vi "Create Session.vi"(8 "error in (no error)":errorcluster, 11 "Session Id":u64) -> (0 "error out":errorcluster, 1 "Run Time Configuration":string, 2 "Edit Time Configuration":string, 3 "Session out":refnum<class "Plugin Session.lvclass">, 4 "Panel Size":T1)   [LabVIEW 2020, in "InstrumentStudio Plugin SDK.lvlib" / "Plugin Session.lvclass"]
doc: "Call this VI with the Session Id as the first SDK call at the beginning of your plugin VI. This VI sets up the events and other data needed for the plugin panel and framework to communicate. If you need to know the panel size for your plugin panel to adjust its front panel, this VI will return the size. Some plugin panels support both large and small panel sizes and need to adjust the visuals on their front panel to better fit into that panel size. LabVIEW plugin panels are uniquely identified by the Plugin Session which is set by the framework when the plugin is run. Plugins must have a control named 'Session Id' which is a U64 numeric control on their plugin VI front panel so the framework can correctly set it. This 'Session Id' is then passed to Create Session.vi to begin the plugin session. This control can be placed on the user's VI by right-clicking on the input of the Create Session.vi and choosing 'Create Control'.\nThe Plugin Session returned is then used to call other SDK VIs during execution of the plugin VI to get or set properties of the plugin panel or to notify the framework of various events."
uses:
  Plugin Session.lvclass
  Panel Size.ctl
  Plugin Events.ctl
  Event Registration Refnum.ctl
  Plugin Session.lvclass/Plugin Session.ctl
  Read Edit Time Configuration.vi
  Read Run Time Configuration.vi
  InstrumentStudio Plugin SDK.lvlib
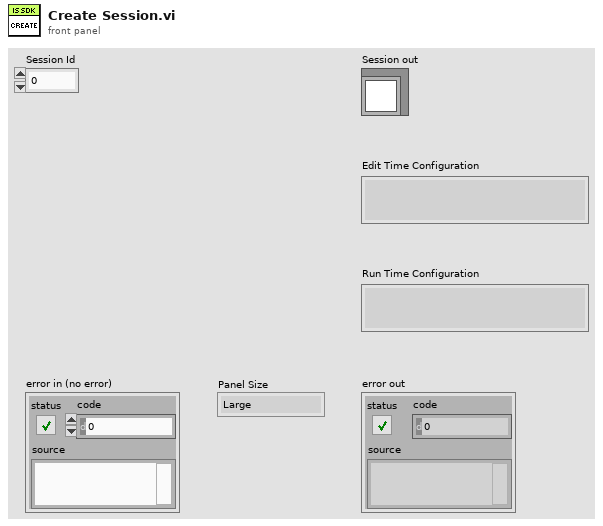
[diagram p1: front panel]
types:
  T1 = typedef "InstrumentStudio Plugin SDK.lvlib/Panel Size.ctl" = enum32{"Large", "Small"}
  T2 = typedef "InstrumentStudio Plugin SDK.lvlib/Plugin Events.ctl" = cluster{"Shutdown":refnum<user-event>, "Project Saved":refnum<user-event>, "Stop All Outputs":refnum<user-event>, "Generic Message":refnum<user-event>, "Active Pin Map Changed":refnum<user-event>, "Selected Sites Changed":refnum<user-event>}
  T3 = typedef "InstrumentStudio Plugin SDK.lvlib/Event Registration Refnum.ctl" = refnum<event-registration>
  T4 = cluster{"Session Id":u64, "Plugin Events":T2, "Event Refnum":T3}
  T5 = cluster{"Active Pin Map Path":path, "Completion Id":i64}
  T6 = cluster{"Name":string, "Data":string, "Completion Id":i64}
  T7 = cluster{"Project Path":path, "Completion Id":i64}
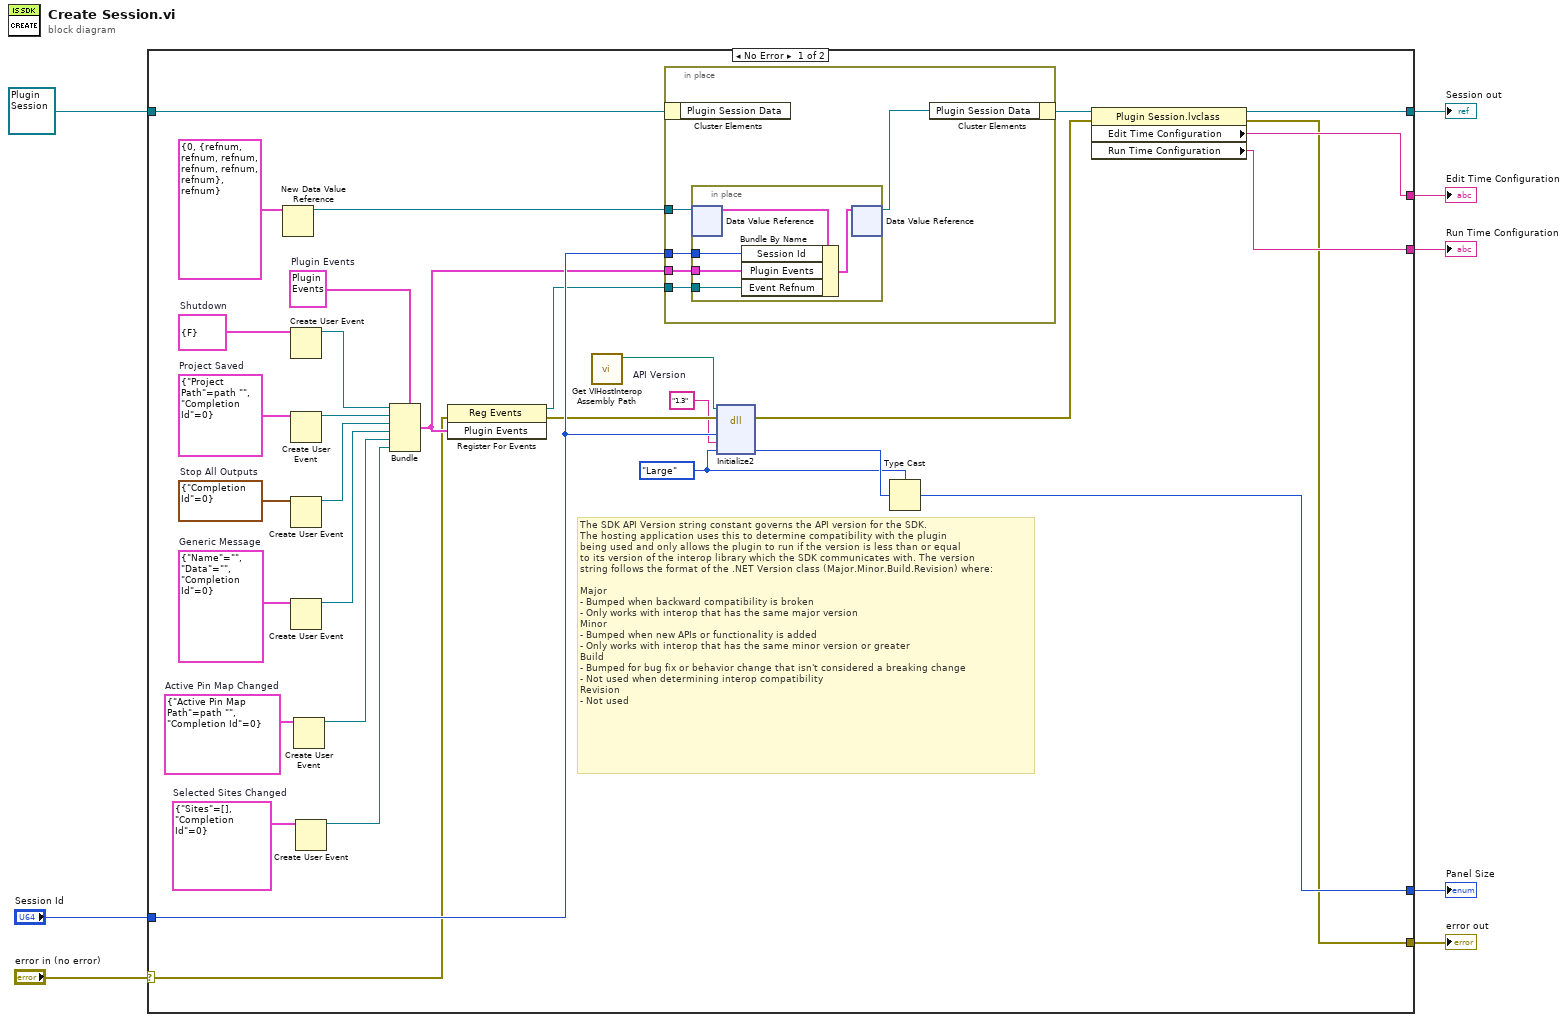
[diagram p0: block diagram]
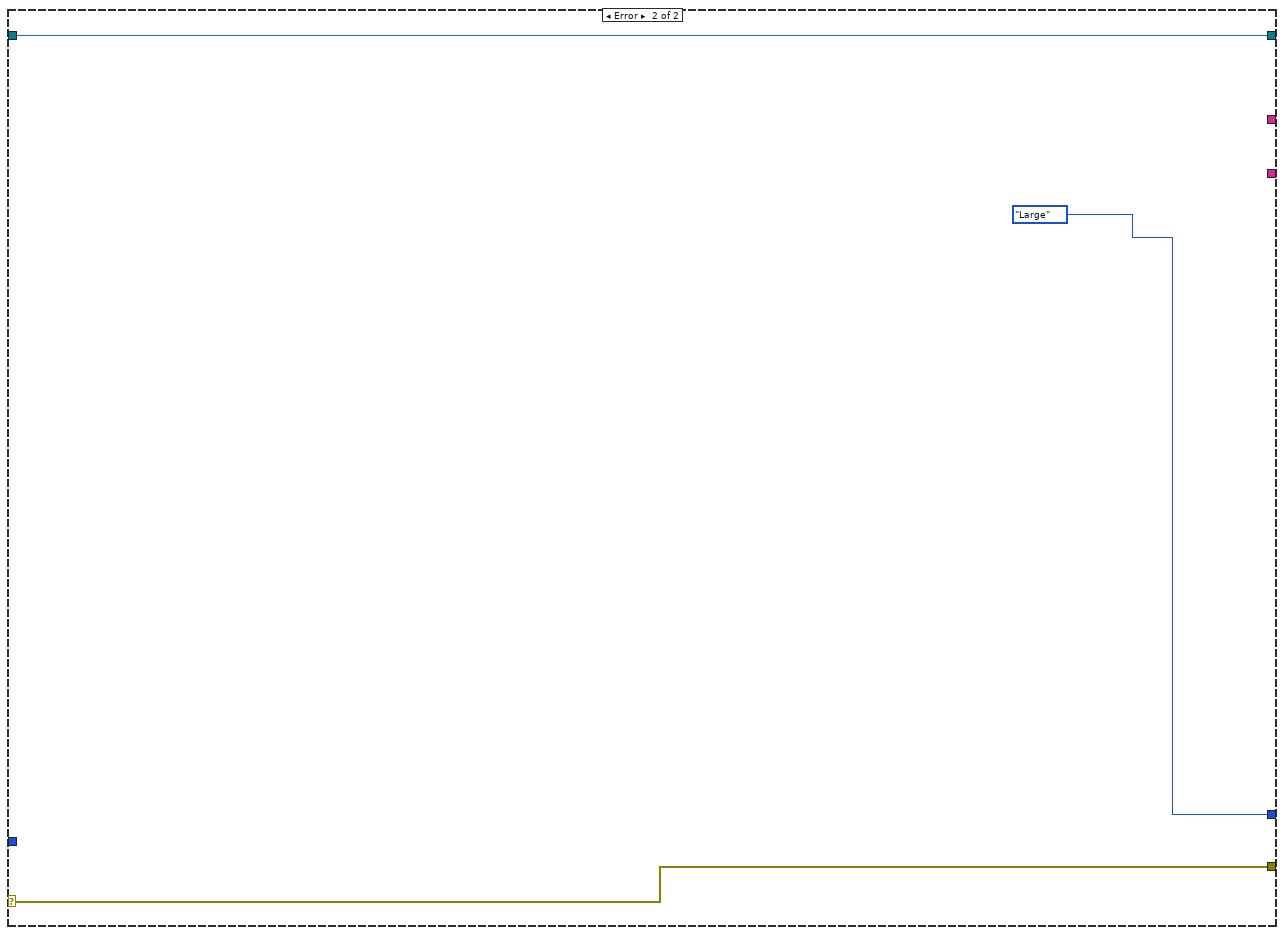
[diagram p2: hidden frame]
diagram:
  n1 = case shown="No Error" "error in (no error)" {
    selector: "error in (no error)" -> [w29 w52]
    tunnel: [w23 w52] -> w8
    tunnel: [w38 Panel_Size."Large" ("Panel Size")] -> w7
    tunnel: "Session Id" -> [w34 _]
    tunnel: refnum<class "Plugin Session.lvclass"> refnum ("PluginSDK:PluginSession.lvclass") -> [w31 w51]
    tunnel: [w24 w51] -> w3
    tunnel: [w27 _] -> w2
    tunnel: [w25 _] -> w1
    frame No Error {
      w13 = cluster{"Sites":i32[], "Completion Id":i64} {"Sites"=[], "Completion Id"=0}  # Selected Sites Changed
      w14 = T5 {"Active Pin Map Path"=path "", "Completion Id"=0}  # Active Pin Map Changed
      w15 = "1.3"  # API Version
      w17 = T6 {"Name"="", "Data"="", "Completion Id"=0}  # Generic Message
      w21 = cluster{"Unused":bool} {"Unused"=FALSE}  # Shutdown
      w12 = T2 {"Shutdown"=refnum, "Project Saved"=refnum, "Stop All Outputs"=refnum, "Generic Message"=refnum, "Active Pin Map Changed"=refnum, "Selected Sites Changed"=refnum}  # Plugin Events
      w36 = T7 {"Project Path"=path "", "Completion Id"=0}  # Project Saved
      w37 = cluster{"Completion Id":i64} {"Completion Id"=0}  # Stop All Outputs
      w39 = Panel_Size."Large" ("Panel Size")
      # "The SDK API Version string constant governs the API version for the SDK.\nThe hosting application uses this to determine compatibility with the plugin\nbeing used and only allows the plugin to run if the version is less than or equal\nto its version of the interop library which the SDK communicates with. The version\nstring follows the format of the .NET Version class (Major.Minor.Build.Revision) where:\n\nMajor\n- Bumped when backward compatibility is broken\n- Only works with interop that has the same major version\nMinor\n- Bumped when new APIs or functionality is added\n- Only works with interop that has the same minor version or greater\nBuild\n- Bumped for bug fix or behavior change that isn't considered a breaking change\n- Not used when determining interop compatibility\nRevision\n- Not used"
      n2 = New Data Value Reference(data value=T4 {"Session Id"=0, "Plugin Events"={"Shutdown"=refnum, "Project Saved"=refnum, "Stop All Outputs"=refnum, "Generic Message"=refnum, "Active Pin Map Changed"=refnum, "Selected Sites Changed"=refnum}, "Event Refnum"=refnum} ("Cluster of class private data")) -> (data value reference=w35:refnum<data-value>)  [unwired: 1 in, 1 out]
      n3 = Create User Event(user event datatype=w21) -> (user event=w20:refnum<user-event>)  [unwired: 1 in, 1 out]
      n4 = Create User Event(user event datatype=w36) -> (user event=w19:refnum<user-event>)  [unwired: 1 in, 1 out]
      n5 = Create User Event(user event datatype=w37) -> (user event=w18:refnum<user-event>)  [unwired: 1 in, 1 out]
      n6 = Create User Event(user event datatype=w17) -> (user event=w16:refnum<user-event>)  [unwired: 1 in, 1 out]
      n7 = Create User Event(user event datatype=w14) -> (user event=w11:refnum<user-event>)  [unwired: 1 in, 1 out]
      n8 = Create User Event(user event datatype=w13) -> (user event=w10:refnum<user-event>)  [unwired: 1 in, 1 out]
      n9 = Bundle(cluster=w12, "Shutdown"=w20, "Project Saved"=w19, "Stop All Outputs"=w18, "Generic Message"=w16, "Active Pin Map Changed"=w11, "Selected Sites Changed"=w10) -> (w33:T2)
      n10 = register-events(error in=w29, w33) -> (reference out=w32:refnum<event-registration>, error out=w30:errorcluster)  [unwired: 1 in]
      n11 = call "Get VIHostInterop Assembly Path.vi"() -> ("VIHost.Interop Assembly"=w9:path)  [unwired: 11 in]
      n12 = in-place {
        in-place-border: w35 -> [w45]
        in-place-border: w34 -> [w44]
        in-place-border: w33 -> [w43]
        in-place-border: w32 -> [w42]
        n13 = in-place-cluster #1(w31) -> ()  [unwired: 1 out]
        n14 = in-place {
          in-place-border: w44 -> [w49]
          in-place-border: w43 -> [w48]
          in-place-border: w42 -> [w47]
          n15 = in-place-dvr #2(w45) -> (w50:T4)  [unwired: 1 out]
          n16 = Bundle By Name(cluster=w50, "Session Id"=w49, "Plugin Events"=w48, "Event Refnum"=w47) -> (w46:T4)
          n17 = in-place-dvr #2(w46) -> (w41:refnum<data-value>)  [unwired: 1 out]
        }
        n18 = in-place-cluster #1("Plugin Session Data"=w41) -> (w26:refnum<class "Plugin Session.lvclass">)
      }
      n19 = dll-call lib="C:/ASW/Source/InstrumentStudio/IFDistribution/VIHostPanel/objects/export/targets/win64U/x64/msvc-14.0/debug/NationalInstruments.VIHost.Interop.dll" fn="Initialize2"(path in=w9, error in=w30, "hostId"=w34, "sdkVersion"=w15, "panelSize"=w39) -> (error out=w22:errorcluster, "panelSize"=w40:u32)  [unwired: 4 in, 1 out]
      n20 = Type Cast(type=w39, x=w40) -> (*(type *) &x=w38:T1)
      n21 = property class="Plugin Session.lvclass"(reference=w26, error in=w22) -> (reference out=w24:refnum<class "Plugin Session.lvclass">, error out=w23:errorcluster, "Edit Time Configuration"=w27:string, "Run Time Configuration"=w25:string)
    }
    frame Error {
    }
  }
  "error out" <- w8
  "Panel Size" <- w7
  "Session out" <- w3
  "Edit Time Configuration" <- w2
  "Run Time Configuration" <- w1
